vi "h.COMM.Read Response.vi"(0 "Connection ID":refnum<k5>, 3 "Timeout":i32=10000, 7 "error in":errorcluster) -> (20 "Connection ID":refnum<k5>, 21 "Status":T2, 22 "Request Option Echo":T1=enum."Suppress Message", 23 "Content Length":u32, 24 "Message Length":u16, 25 "Content":u8[](array[numeric]), 26 "Message":string, 27 "error out":errorcluster)   [LabVIEW 2019, in "h.Library.lvlib"]
doc: "This vi is invoked following a call to the h.COMM.Write Command.vi to retrieve the response to the executed command.\n\nThis vi sends a command and argument to a Hyperion instrument.\n\n<b>Connection ID</b> - is a network connection refnum that uniquely identifies the TCP connection\n<b>Timeout</b> - specifies the maximum amount of time, in milliseconds, for the function to complete\n<b>error in</b> - describes error conditions that occur before this node runs. This input provides standard error functionality\n<b>Connection ID out</b> - Returns the same value as connection ID\n<b>Type</b> - The type of the retured response\n<b>Message</b> - human readable message providing info on the status of the executed command\n<b>Message Length</b> - byte length of the returned <b>Message</b>\n<b>Content</b> - the content of the returned command\n<b>Content Length</b> - the length of the returned <b>Content</b>s\n<b>error out</b> - contains error information. This output provides standard error out functionality."
uses:
  h.Library.lvlib
  CTL/h.COMM.Command Status Enum.ctl
  CTL/h.COMM.RequestCommandOptions.ctl
  CTL/h.COMM.Command Response Cluster.ctl
panel:
  # "Hyperion Read Command Response"
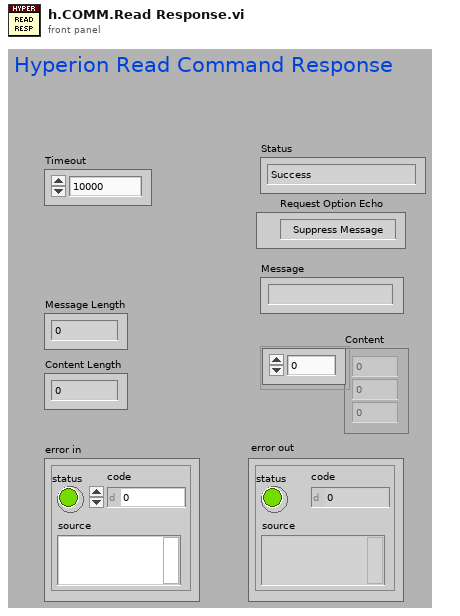
[diagram p1: front panel]
types:
  T1 = typedef "h.Library.lvlib/h.COMM.RequestCommandOptions.ctl" = enum8{"None", "Suppress Message", "Suppress Content", "Compress"}
  T2 = typedef "h.Library.lvlib/h.COMM.Command Status Enum.ctl" = enum8{"Success", "Failed", "Error", "AccessDenied", "InvalidCommand", "InvalidNumberArguments", "InvalidArgument", ""}
  T3 = typedef "h.Library.lvlib/h.COMM.Command Response Cluster.ctl" = cluster{"Content Length":u32, "Message Length":u16, "Request Option Echo":T1, "Status":T2}
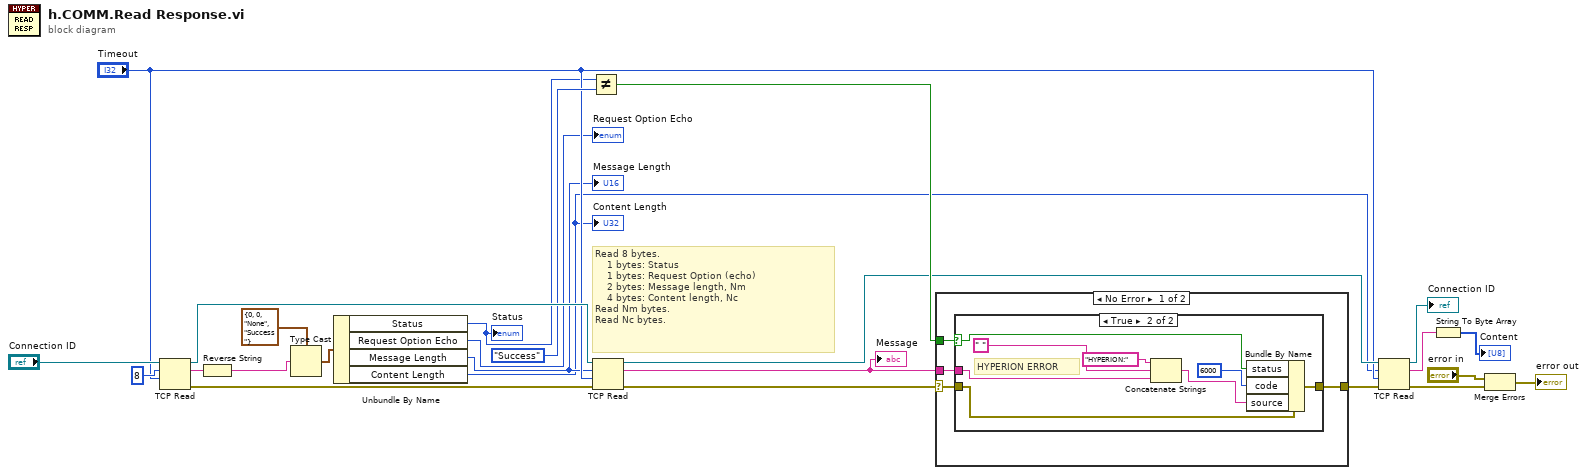
[diagram p0: block diagram]
diagram:
  # "Read 8 bytes.\n    1 bytes: Status\n    1 bytes: Request Option (echo)\n    2 bytes: Message length, Nm\n    4 bytes: Content length, Nc\nRead Nm bytes.\nRead Nc bytes."
  n1 = TCP Read(connection ID="Connection ID", bytes to read=8, 9:"Timeout") -> (connection ID out=w22:refnum<k5>, data out=w5:string, error out=w24:errorcluster)  [unwired: 2 in]
  n2 = Reverse String(1:w5) -> (0:w4:string)
  n3 = Type Cast(type=T3 {"Content Length"=0, "Message Length"=0, "Request Option Echo"=enum."None", "Status"=enum."Success"} ("Command Response"), x=w4) -> (*(type *) &x=w19:T3)
  n4 = Unbundle By Name(w19) -> ("Status"=w9:T2, "Request Option Echo"=→"Request Option Echo":T1, "Message Length"=w7:u16, "Content Length"=w6:u32)
  "Content Length" <- w6
  "Status" <- w9
  "Message Length" <- w7
  n5 = Not Equal?(x=w9, y=h.COMM.Command_Status_Enum."Success") -> (x != y?=w17:bool)
  n6 = TCP Read(connection ID=w22, bytes to read=w7, error in (no error)=w24, 9:"Timeout") -> (connection ID out=w15:refnum<k5>, data out=w16:string, error out=w20:errorcluster)  [unwired: 1 in]
  "Message" <- w16
  n7 = case shown="No Error" w20 {
    selector: w20 -> [w28 w39]
    tunnel: w17 -> [w29 _]
    tunnel: [w27 w39] -> w14
    tunnel: w16 -> [w26 _]
    frame No Error {
      n8 = case shown="True" w29 {
        selector: w29 -> [_ w37]
        tunnel: w28 -> [w30 w38]
        tunnel: [w30 w36] -> w27
        tunnel: w26 -> [_ w31]
        frame False {
          # "NO ERROR"
        }
        frame True {
          # "HYPERION ERROR"
          n9 = Concatenate Strings("HYPERION:" ("source"), " ", w31) -> (w34:string)
          n10 = Bundle By Name(cluster=w38, "status"=w37, "code"=6000, "source"=w34) -> (w36:errorcluster)
        }
      }
    }
    frame Error {
      # "System (Not HYPERION) Error"
    }
  }
  n11 = TCP Read(connection ID=w15, bytes to read=w6, error in (no error)=w14, 9:"Timeout") -> (connection ID out=→"Connection ID":refnum<k5>, data out=w13:string, error out=w2:errorcluster)  [unwired: 1 in]
  n12 = String To Byte Array(string=w13) -> (unsigned byte array=→"Content":u8[])
  n13 = Merge Errors("error in", w2) -> (→"error out":errorcluster)
